vi "通道字符串转换数值常量2.vi"(1 "?":string(combo)) -> (0 "数值":i32)   [LabVIEW 2014]
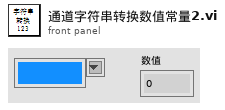
[diagram p1: front panel]
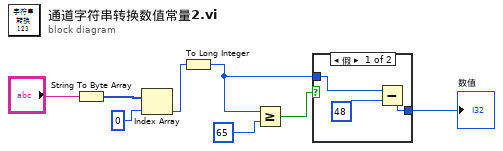
[diagram p0: block diagram]
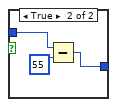
[diagram p2: hidden frame]
diagram:
  n1 = String To Byte Array(string="?") -> (unsigned byte array=w7:u8[])
  n2 = Index Array(array=w7, index=0) -> (element=w2:u8)
  n3 = To Long Integer(number=w2) -> (32bit integer=w1:i32)
  n4 = Greater Or Equal?(x=w1, y=65) -> (x >= y?=w5:bool)
  n5 = case shown="假" w5 {
    tunnel: w1 -> [w10 w14]
    tunnel: [w9 w12] -> w3
    frame False {
      n6 = Subtract(x=w10, y=48) -> (x-y=w9:i32)
    }
    frame True {
      n7 = Subtract(x=w14, y=55) -> (x-y=w12:i32)
    }
  }
  "数值" <- w3
